vi "Check Message Occurrences.vi"(8 "error in (no error)":errorcluster, 10 "Message":string) -> (0 "error IO":errorcluster, 2 "Occurences":i32)   [LabVIEW 2018, in "Instrument Addon Common System Tests.lvclass"]
uses:
  Instrument Addon Common System Tests.lvclass
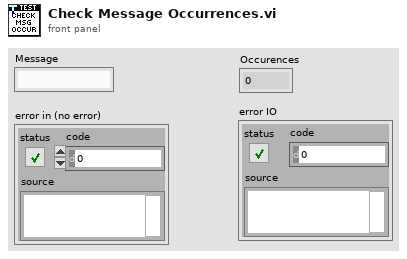
[diagram p1: front panel]
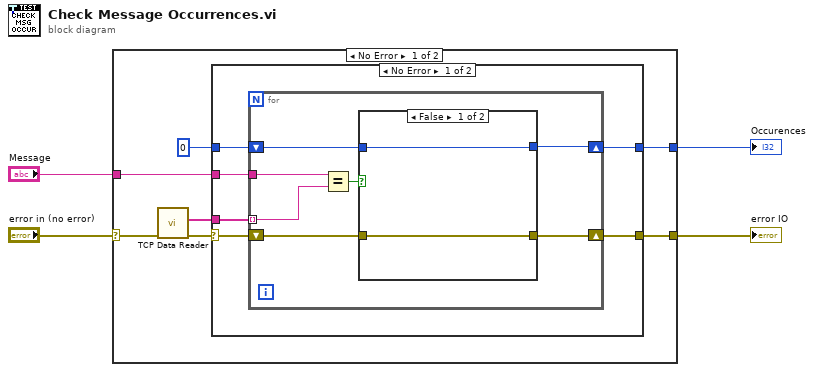
[diagram p0: block diagram]
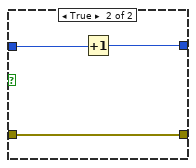
[diagram p2: hidden frame]
diagram:
  n1 = case shown="No Error" "error in (no error)" {
    selector: "error in (no error)" -> [w8 w32]
    tunnel: "Message" -> [w10 _]
    tunnel: [w6 w32] -> w1
    tunnel: [w5 _] -> w2
    frame No Error {
      n2 = call "TCP Data Reader.vi"("error in (no error)"=w8) -> ("error out"=w7:errorcluster, "Recieved Messages"=w9:string[])  [unwired: 8 in, 1 out]
      n3 = case shown="No Error" w7 {
        selector: w7 -> [w14 w31]
        tunnel: 0 -> [w17 w30]
        tunnel: w10 -> [w16 _]
        tunnel: w9 -> [w15 _]
        tunnel: [w13 w31] -> w6
        tunnel: [w12 w30] -> w5
        frame No Error {
          n4 = for {
            tunnel: w15 -> [w21] mode=indexing
            tunnel: w16 -> [w20]
            shift-right: [w22] -> w12
            shift-left: w17 -> [w23]
            shift-right: [w18] -> w13
            shift-left: w14 -> [w19]
            n5 = Equal?(x=w20, y=w21) -> (x = y?=w24:bool)
            n6 = case shown="False" w24 {
              tunnel: w23 -> [w26 w29]
              tunnel: [w26 w28] -> w22
              tunnel: w19 -> [w25 w27]
              tunnel: [w25 w27] -> w18
              frame False {
              }
              frame True {
                n7 = Increment(x=w29) -> (x+1=w28:i32)
              }
            }
          }
        }
        frame Error {
        }
      }
    }
    frame Error {
    }
  }
  "Occurences" <- w2
  "error IO" <- w1
